vi "Double_GeneralGearShift_WithDeadTime_4Mtr.vi"(6 "error In":errorcluster, 7 "ShifterRef":T1={"DevStatus"={"status"=FALSE, "code"=0, "source"=""}, "Pneumatics Control Module"=0, "Forward Solenoid Channel"=enum."Invalid", "Reverse Solenoid Channel"=enum."Invalid"}, 9 "Shift Value":T3, 10 "Right":dbl, 11 "Left":dbl) -> (0 "error out":errorcluster, 1 "Shifting":bool, 2 "Right Output":dbl, 3 "Left Output":dbl)   [LabVIEW 2017]
uses:
  <vilib>/Rock Robotics/WPI/Solenoid/WPI_SolenoidValue.ctl
  <vilib>/Rock Robotics/WPI/Solenoid/WPI_SolenoidDevRef.ctl
  <vilib>/Rock Robotics/WPI/Solenoid/WPI_SolenoidChannel.ctl
  <vilib>/Rock Robotics/WPI/ThirdParty/Phoenix-LabVIEW/Motor Controller/Controls/CTRE_Phoenix_MotorControl_NeutralMode.ctl
  <vilib>/Rock Robotics/WPI/Solenoid/WPI_SolenoidSetEnum.vi
panel:
  out "Right Setpoint":dbl
  out "Left Setpoint":dbl
  out "TempTimeVal":u32
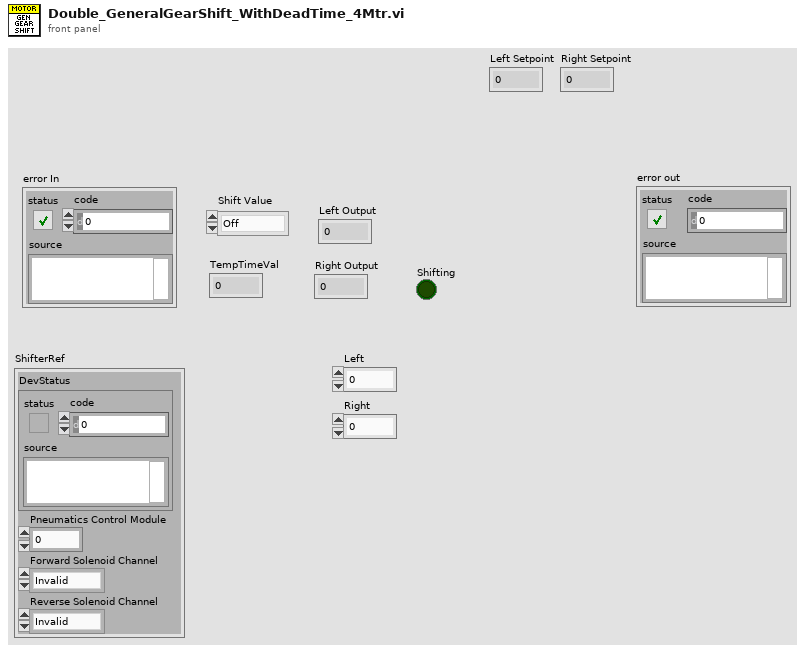
[diagram p1: front panel]
types:
  T1 = typedef "WPI_SolenoidDevRef.ctl" = cluster{"DevStatus":errorcluster, "Pneumatics Control Module":u8, "Forward Solenoid Channel":T2, "Reverse Solenoid Channel":T2}
  T2 = typedef "WPI_SolenoidChannel.ctl" = enum8{"Solenoid 0", "Solenoid 1", "Solenoid 2", "Solenoid 3", "Solenoid 4", "Solenoid 5", "Solenoid 6", "Solenoid 7", "Invalid"}
  T3 = typedef "WPI_SolenoidValue.ctl" = enum16{"Off", "On", "Forward", "Reverse"}
  T4 = typedef "WPI_MotorControlDeviceRef.ctl" = cluster{"DeviceStatus":errorcluster, "Type":T5, "PWM":cluster{"PWM Channel":T6, "DeadBand":T7}, "CAN":cluster{"Device Number":u8, "SetOutput VI Ref":variant, "GetOutput VI Ref":variant, "Enable VI Ref":variant, "Disable VI Ref":variant, "Data":variant}, "Invert":bool, "DIO PWM":cluster{"PWM \"Enable\" Channel":T6, "DIOChannel":T8, "PWM Rate":dbl}}
  T5 = typedef "WPI_MotorControlType.ctl" = enum16{"PWM", "CAN", "DIO PWM"}
  T6 = typedef "FPGA_DIOPWMChannel.ctl" = enum8{"PWM 0", "PWM 1", "PWM 2", "PWM 3", "PWM 4", "PWM 5", "PWM 6", "PWM 7", "PWM 8", "PWM 9", "PWM MXP 0", "PWM MXP 1", "PWM MXP 2", "PWM MXP 3", "PWM MXP 4", "PWM MXP 5", "PWM MXP 6", "PWM MXP 7", "PWM MXP 8", "PWM MXP 9", "Invalid"}
  T7 = typedef "WPI_PWMDeadband.ctl" = cluster{"Name":string, "maxPositivePwm":i32, "minPositivePwm":i32, "centerPwm":i32, "maxNegativePwm":i32, "minNegativePwm":i32, "angularRange":u16}
  T8 = typedef "FPGA_DIOChannel.ctl" = enum8{"DIO 0", "DIO 1", "DIO 2", "DIO 3", "DIO 4", "DIO 5", "DIO 6", "DIO 7", "DIO 8", "DIO 9", "DIO MXP 0", "DIO MXP 1", "DIO MXP 2", "DIO MXP 3", "DIO MXP 4", "DIO MXP 5", "DIO MXP 6", "DIO MXP 7", "DIO MXP 8", "DIO MXP 9", "DIO MXP 10", "DIO MXP 11", "DIO MXP 12", "DIO MXP 13", "DIO MXP 14", "DIO MXP 15", "SPI Port CS1", "SPI Port CS2", "SPI Port CS3", "SPI Port MISO", "SPI Port MOSI", "Invalid"}
  T9 = typedef "CTRE_Phoenix_MotorControl_NeutralMode.ctl" = enum8{"EEPROMSetting", "Override to Coast", "Override to Brake"}
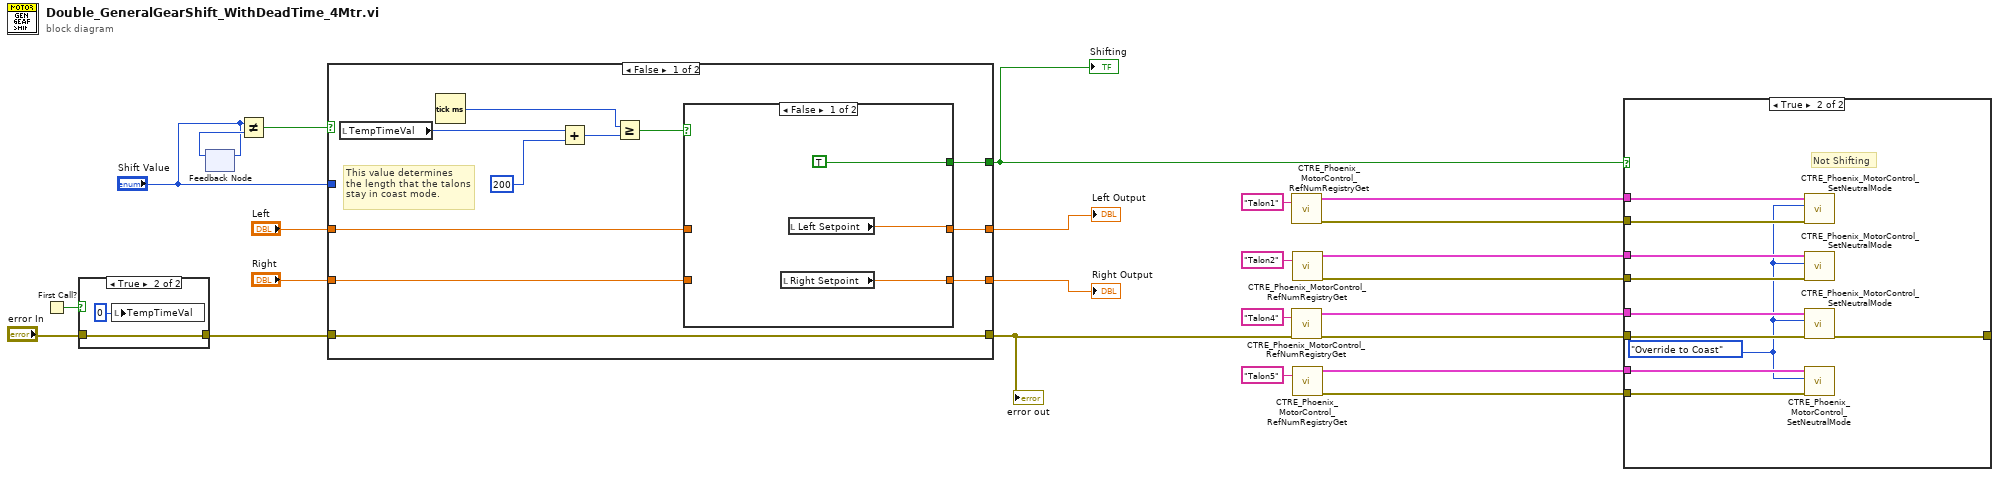
[diagram p0: block diagram]
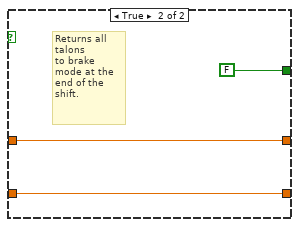
[diagram p4: hidden frame]
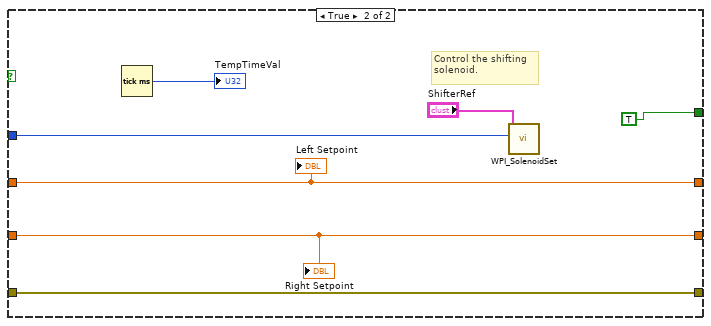
[diagram p5: hidden frame]
diagram:
  n1 = First Call?() -> (First Call?: T/F=w20:bool)
  n2 = case shown="True" w20 {
    tunnel: [w25 w26] -> w15
    tunnel: "error In" -> [w25 w26]
    frame False {
    }
    frame True {
      n3 = local write "TempTimeVal"(u32 0 ("TempTimeVal")) -> ()
    }
  }
  n4 = feedback-in #1("Shift Value") -> ()
  n5 = feedback #1() -> (w18:T3)  [unwired: 1 in]
  n6 = Not Equal?(x="Shift Value", y=w18) -> (x != y?=w17:bool)
  n7 = case shown="False" w17 {
    tunnel: [w38 w46] -> w24
    tunnel: [w37 w45] -> w23
    tunnel: "Right" -> [w36 w45]
    tunnel: "Left" -> [w35 w46]
    tunnel: [w29 TRUE] -> w1
    tunnel: "Shift Value" -> [_ w48]
    tunnel: w15 -> [w28 w47]
    tunnel: [w28 w47] -> w14
    frame False {
      # "This value determines\nthe length that the talons\nstay in coast mode."
      n8 = local read "TempTimeVal"() -> (w31:u32)
      n9 = Tick Count (ms)() -> (millisecond timer value=w33:u32)
      n10 = Add(x=w31, y=200) -> (x+y=w32:u32)
      n11 = Greater Or Equal?(x=w33, y=w32) -> (x >= y?=w34:bool)
      n12 = case shown="False" w34 {
        tunnel: [w39 w43] -> w38
        tunnel: [w40 w44] -> w37
        tunnel: w36 -> [_ w44]
        tunnel: w35 -> [_ w43]
        tunnel: [TRUE FALSE] -> w29
        frame False {
          n13 = local read "Right Setpoint"() -> (w40:dbl)
          n14 = local read "Left Setpoint"() -> (w39:dbl)
        }
        frame True {
          # "Returns all talons\nto brake mode at the\nend of the shift."
        }
      }
    }
    frame True {
      # "Control the shifting\nsolenoid."
      n15 = Tick Count (ms)() -> (millisecond timer value=→"TempTimeVal":u32)
      n16 = call-poly <vilib>:"WPI_SolenoidSet.vi"("Value"=w48, "SolenoidDevRef"="ShifterRef") -> ()  [unwired: 8 in, 2 out]
      "Left Setpoint" <- w46
      "Right Setpoint" <- w45
    }
  }
  "Left Output" <- w24
  "Right Output" <- w23
  "error out" <- w14
  "Shifting" <- w1
  n17 = call <vilib>:"CTRE_Phoenix_MotorControl_RefNumRegistryGet.vi"("refnum name"="Talon1") -> ("error out"=w8:errorcluster, "PhoenixMotorControlDevRef"=w9:T4)  [unwired: 9 in]
  n18 = call <vilib>:"CTRE_Phoenix_MotorControl_RefNumRegistryGet.vi"("error in (no error)"=w14, "refnum name"="Talon4") -> ("error out"=w4:errorcluster, "PhoenixMotorControlDevRef"=w5:T4)  [unwired: 8 in]
  n19 = call <vilib>:"CTRE_Phoenix_MotorControl_RefNumRegistryGet.vi"("refnum name"="Talon2") -> ("error out"=w6:errorcluster, "PhoenixMotorControlDevRef"=w7:T4)  [unwired: 9 in]
  n20 = call <vilib>:"CTRE_Phoenix_MotorControl_RefNumRegistryGet.vi"("refnum name"="Talon5") -> ("error out"=w2:errorcluster, "PhoenixMotorControlDevRef"=w3:T4)  [unwired: 9 in]
  n21 = case shown="True" w1 {
    tunnel: w9 -> [_ w62]
    tunnel: w8 -> [_ w61]
    tunnel: w7 -> [_ w60]
    tunnel: w6 -> [_ w59]
    tunnel: w4 -> [w52 w57]
    tunnel: w5 -> [_ w58]
    tunnel: w3 -> [_ w56]
    tunnel: w2 -> [_ w55]
    tunnel: [w52 w53] -> _
    frame False {
    }
    frame True {
      w54 = CTRE_Phoenix_MotorControl_NeutralMode."Override to Coast" ("Motor Control Neutral Mode")
      # "Not Shifting"
      n22 = call <vilib>:"CTRE_Phoenix_MotorControl_SetNeutralMode.vi"("error in (no error)"=w61, "Motor Control Neutral Mode"=w54, "PhoenixMotorControlDevRef"=w62) -> ()  [unwired: 7 in, 2 out]
      n23 = call <vilib>:"CTRE_Phoenix_MotorControl_SetNeutralMode.vi"("error in (no error)"=w59, "Motor Control Neutral Mode"=w54, "PhoenixMotorControlDevRef"=w60) -> ()  [unwired: 7 in, 2 out]
      n24 = call <vilib>:"CTRE_Phoenix_MotorControl_SetNeutralMode.vi"("error in (no error)"=w57, "Motor Control Neutral Mode"=w54, "PhoenixMotorControlDevRef"=w58) -> ("error out"=w53:errorcluster)  [unwired: 7 in, 1 out]
      n25 = call <vilib>:"CTRE_Phoenix_MotorControl_SetNeutralMode.vi"("error in (no error)"=w55, "Motor Control Neutral Mode"=w54, "PhoenixMotorControlDevRef"=w56) -> ()  [unwired: 7 in, 2 out]
    }
  }
